vi "Construct (Range).vi"(8 "Error in (no error)":errorcluster, 9 "Priority Lower":T1 items=["EMERGENCY", "ALERT", "CRITICAL", "ERROR", "WARNING", "NOTICE", "INFO", "DEBUG"], 10 "Priority Upper":T1 items=["EMERGENCY", "ALERT", "CRITICAL", "ERROR", "WARNING", "NOTICE", "INFO", "DEBUG"], 11 "LogFilterPriority in":refnum<class "LogFilterPriority.lvclass">) -> (0 "Error out":errorcluster, 3 "LogFilterPriority out":refnum<class "LogFilterPriority.lvclass">)   [LabVIEW 2011, in "LogFilterPriority.lvclass"]
uses:
  LogFilterPriority.lvclass
  Log/PrioritiesRing.ctl
  LogFilterPriority.lvclass/LogFilterPriority.ctl
  Log/Log.lvclass
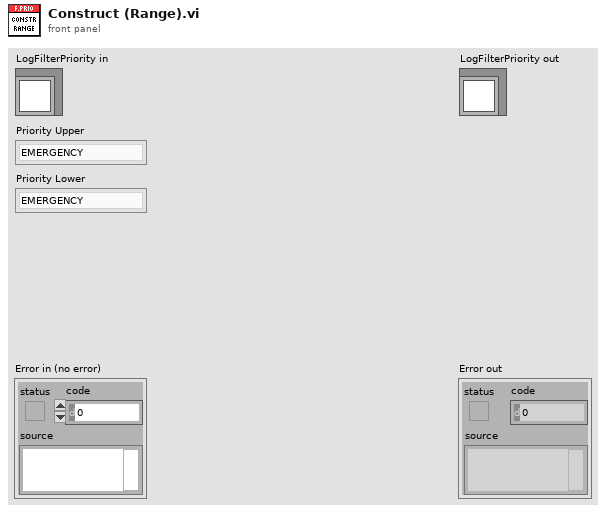
[diagram p1: front panel]
types:
  T1 = typedef "Log.lvclass/PrioritiesRing.ctl" = u32
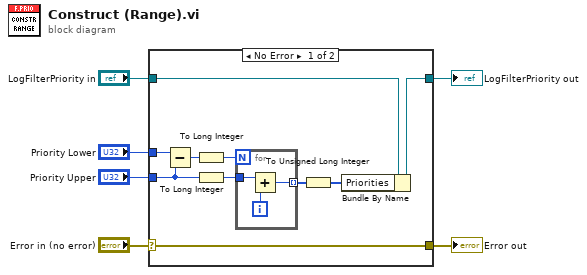
[diagram p0: block diagram]
diagram:
  n1 = case shown="No Error" "Error in (no error)" {
    selector: "Error in (no error)" -> [w16 w21]
    tunnel: [w16 w21] -> w5
    tunnel: [w9 w20] -> w3
    tunnel: "LogFilterPriority in" -> [w11 w20]
    tunnel: "Priority Upper" -> [w7 _]
    tunnel: "Priority Lower" -> [w8 _]
    frame No Error {
      n2 = Subtract(x=w8, y=w7) -> (x-y=w15:T1)
      n3 = To Long Integer(number=w15) -> (32bit integer=w14:i32)
      n4 = To Long Integer(number=w7) -> (32bit integer=w13:i32)
      n5 = for {
        N: w14 -> [_]
        tunnel: w13 -> [w19]
        tunnel: [w17] -> w12 mode=indexing
        i -> [w18]
        n6 = Add(x=w19, y=w18) -> (x+y=w17:i32)
      }
      n7 = To Unsigned Long Integer(number=w12) -> (unsigned 32bit integer=w10:u32[])
      n8 = Bundle By Name(cluster=w11, "Priorities"=w10) -> (w9:refnum<class "LogFilterPriority.lvclass">)
    }
    frame Error {
    }
  }
  "Error out" <- w5
  "LogFilterPriority out" <- w3
